vi "显示一组数据不需要输入结果 - 副本.vi"(6 "Text Color (black)":u32(colorbox)=16860, 8 "显示坐标":cluster{dbl, "Numeric":dbl}[](array[cluster]), 9 "Font, Size & Style":T2={"Desired Font (Application)"=enum."User-specified Font", "[User-specified Font]"={"Font Name"="", "Size"=60, "Strikeout?"=FALSE, "Italic?"=FALSE, "Underline?"=FALSE, "Outline?"=FALSE, "Shadow?"=FALSE, "Bold?"=FALSE, "Rotation Angle"=0.0}, "Horizontal Alignment"=0, "Vertical Alignment"=0} {"Horizontal Alignment" items=["Left", "Center", "Right"]; "Vertical Alignment" items=["Bottom", "Top", "Baseline"]}, 10 "待写入数据":dbl[](array[numeric]), 11 "Img输入":T1) -> (3 "Img输出":T1)   [LabVIEW 2014]
uses:
  <vilib>/vision/Image Controls.llb/IMAQ Image.ctl
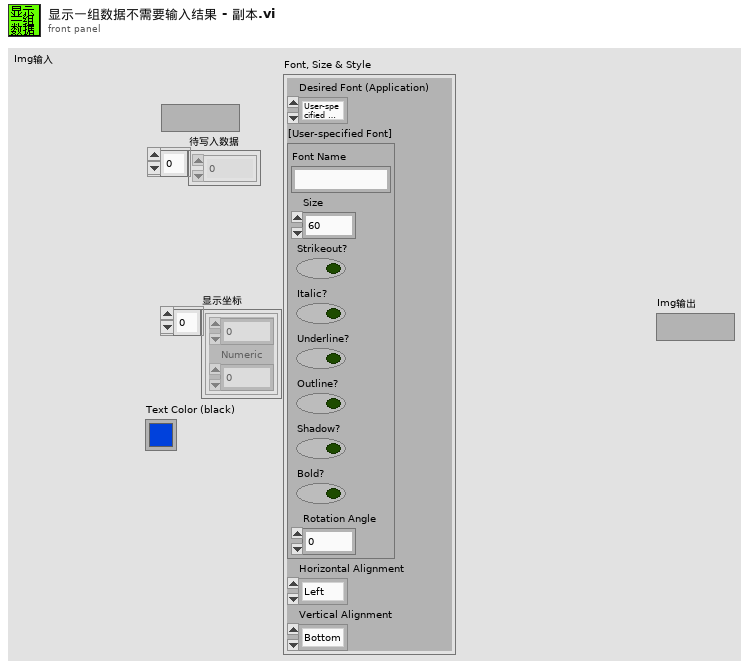
[diagram p1: front panel]
types:
  T1 = typedef "IMAQ Image.ctl" = refnum<image>
  T2 = cluster{"Desired Font (Application)":enum16{"User-specified Font", "Application Font", "System Font", "Dialog Font"}, "[User-specified Font]":cluster{"Font Name":string, "Size":i16, "Strikeout?":bool, "Italic?":bool, "Underline?":bool, "Outline?":bool, "Shadow?":bool, "Bold?":bool, "Rotation Angle":dbl}, "Horizontal Alignment":i16, "Vertical Alignment":i16}
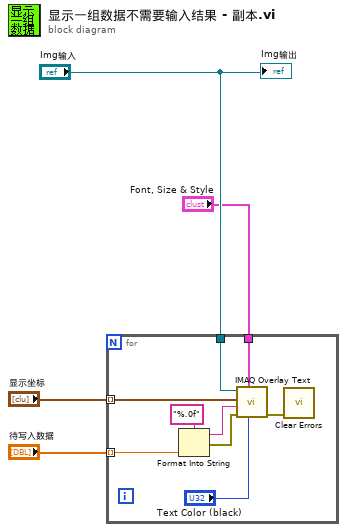
[diagram p0: block diagram]
diagram:
  n1 = for {
    tunnel: "Img输入" -> [w13]
    tunnel: "待写入数据" -> [w12] mode=indexing
    tunnel: "显示坐标" -> [w11] mode=indexing
    tunnel: "Font, Size & Style" -> [w10]
    n2 = Format Into String(format string="%.0f" ("格式字符串"), w12) -> (resulting string=w9:string, error out=w7:errorcluster)  [unwired: 2 in]
    n3 = call "IMAQ Overlay Text"("Text Color (black)"="Text Color (black)", "Font, Size & Style"=w10, "error in (no error)"=w7, "String"=w9, "Origin"=w11, "Image"=w13) -> ("error out"=w6:errorcluster)  [unwired: 4 in, 1 out]
    n4 = call <vilib>:"Clear Errors.vi"("error in (no error)"=w6) -> ()  [unwired: 5 in, 2 out]
  }
  "Img输出" <- "Img输入"
